vi "BDC to BIN.vi"(1 "BDC0":T2, 2 "BDC1":T3) -> (0 "R":T1)   [LabVIEW 2013]
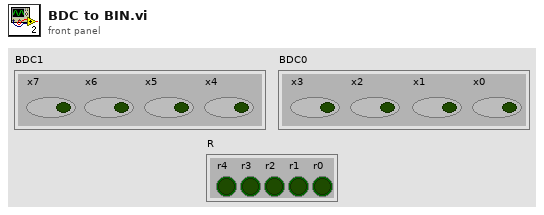
[diagram p1: front panel]
types:
  T1 = cluster{"r4":bool, "r3":bool, "r2":bool, "r1":bool, "r0":bool}
  T2 = cluster{"x3":bool, "x2":bool, "x1":bool, "x0":bool}
  T3 = cluster{"x7":bool, "x6":bool, "x5":bool, "x4":bool}
  T4 = cluster{"x7":bool, "y3":bool, "y3":bool, "y3":bool, "y3":bool}
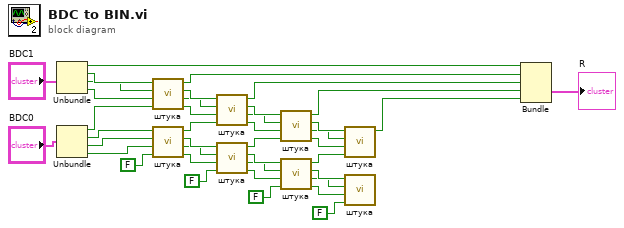
[diagram p0: block diagram]
diagram:
  n1 = Unbundle("BDC1") -> ("x7"=w29:bool, "x6"=w38:bool, "x5"=w37:bool, "x4"=w36:bool)
  n2 = Unbundle("BDC0") -> ("x3"=w35:bool, "x2"=w34:bool, "x1"=w33:bool, "x0"=w32:bool)
  n3 = call "штука.vi"("x0"=w35, "x1"=w36, "x2"=w37, "x3"=w38) -> ("y0"=w25:bool, "y1"=w26:bool, "y2"=w27:bool, "y3"=w28:bool)
  n4 = call "штука.vi"("x0"=FALSE, "x1"=w32, "x2"=w33, "x3"=w34) -> ("y0"=w21:bool, "y1"=w22:bool, "y2"=w23:bool, "y3"=w24:bool)
  n5 = call "штука.vi"("x0"=w24, "x1"=w25, "x2"=w26, "x3"=w27) -> ("y0"=w16:bool, "y1"=w17:bool, "y2"=w18:bool, "y3"=w19:bool)
  n6 = call "штука.vi"("x0"=FALSE, "x1"=w21, "x2"=w22, "x3"=w23) -> ("y0"=w12:bool, "y1"=w13:bool, "y2"=w14:bool, "y3"=w15:bool)
  n7 = call "штука.vi"("x0"=w15, "x1"=w16, "x2"=w17, "x3"=w18) -> ("y0"=w7:bool, "y1"=w8:bool, "y2"=w9:bool, "y3"=w10:bool)
  n8 = call "штука.vi"("x0"=FALSE, "x1"=w12, "x2"=w13, "x3"=w14) -> ("y0"=w3:bool, "y1"=w4:bool, "y2"=w5:bool, "y3"=w6:bool)
  n9 = call "штука.vi"("x0"=w6, "x1"=w7, "x2"=w8, "x3"=w9) -> ("y3"=w1:bool)  [unwired: 3 out]
  n10 = call "штука.vi"("x0"=FALSE, "x1"=w3, "x2"=w4, "x3"=w5) -> ()  [unwired: 4 out]
  n11 = Bundle("x7"=w29, "y3"=w28, "y3"=w19, "y3"=w10, "y3"=w1) -> (→"R":T4)  [unwired: 1 in]
